vi "WS1050_VSA_Convert_Data Updated.vi"(6 "VSA_C3":string[][](array[string]), 7 "WS1050/51":bool=TRUE, 8 "error in (no error)":errorcluster, 9 "VSA_C2":string[][](array[string]), 10 "VSA_C1":string[][](array[string]), 11 "Voltage":string[][](array[string])) -> (0 "error out":errorcluster, 1 "VSA_V3":string[][](array[string]), 2 "VSA_V2":string[][](array[string]), 3 "VSA_V1":string[][](array[string]))   [LabVIEW 2012]
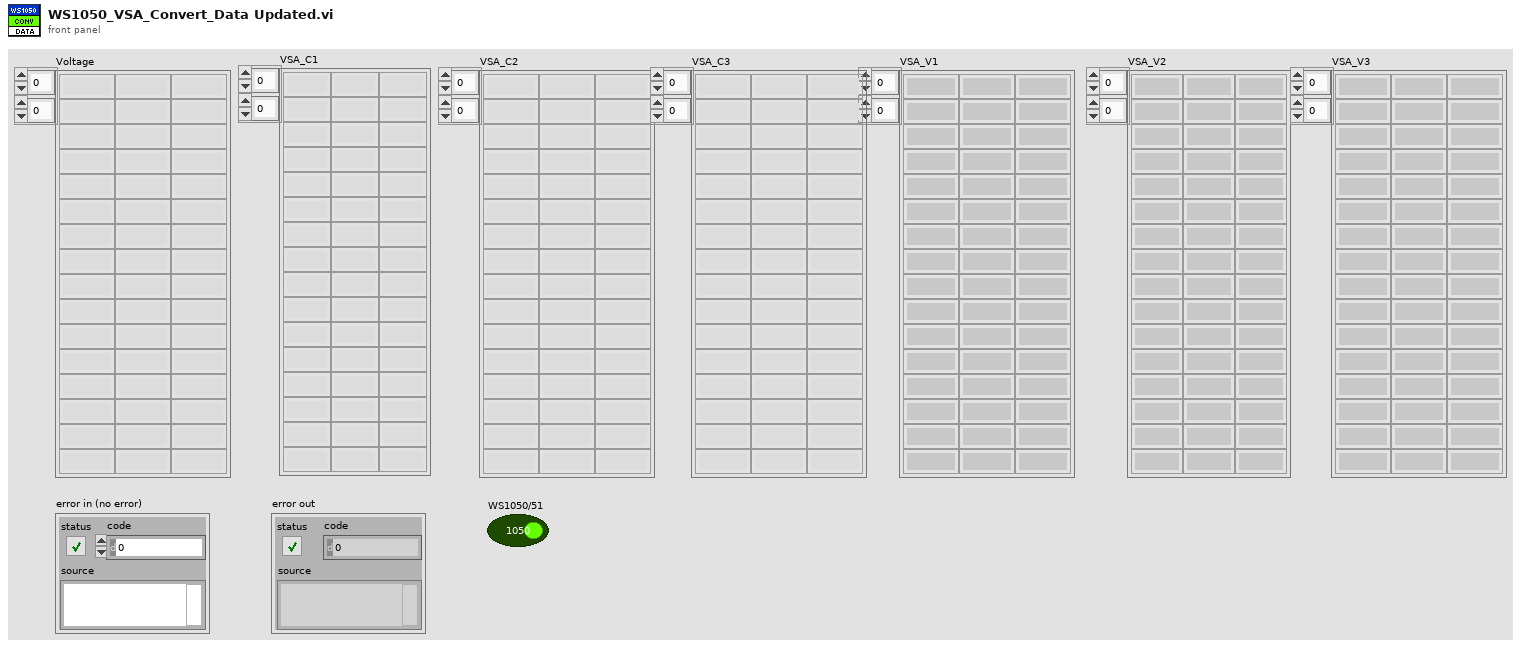
[diagram p1: front panel]
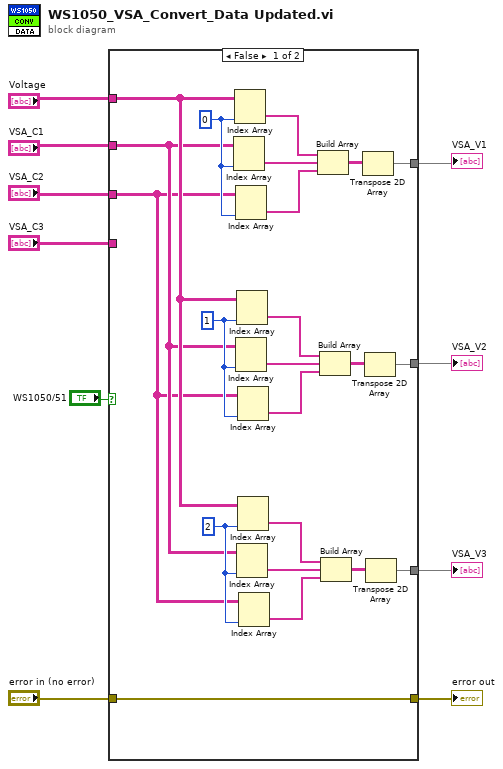
[diagram p0: block diagram]
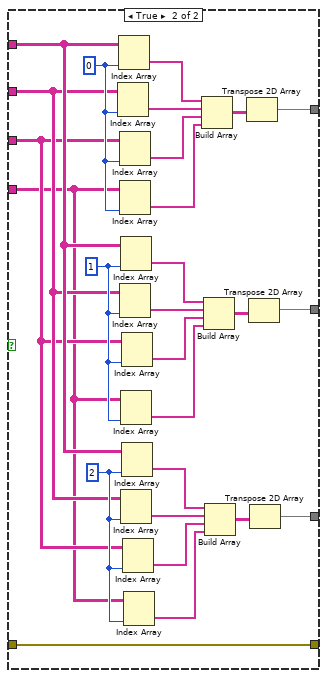
[diagram p2: hidden frame]
diagram:
  n1 = case shown="False" "WS1050/51" {
    tunnel: "error in (no error)" -> [w11 w58]
    tunnel: [w11 w58] -> w9
    tunnel: "Voltage" -> [w16 w57]
    tunnel: "VSA_C1" -> [w15 w38]
    tunnel: "VSA_C2" -> [w14 w37]
    tunnel: "VSA_C3" -> [_ w36]
    tunnel: [w17 w35] -> w3
    tunnel: [w12 w34] -> w2
    tunnel: [w13 w33] -> w1
    frame False {
      w18 = 2 ("disabled index (col)")
      w19 = 1 ("disabled index (col)")
      w20 = 0 ("disabled index (col)")
      n2 = Index Array(array=w15, index (col)=w20) -> (element=w31:string[])  [unwired: 1 in]
      n3 = Index Array(array=w16, index (col)=w20) -> (element=w32:string[])  [unwired: 1 in]
      n4 = Index Array(array=w14, index (col)=w20) -> (element=w30:string[])  [unwired: 1 in]
      n5 = Index Array(array=w15, index (col)=w19) -> (element=w26:string[])  [unwired: 1 in]
      n6 = Index Array(array=w16, index (col)=w19) -> (element=w25:string[])  [unwired: 1 in]
      n7 = Index Array(array=w15, index (col)=w18) -> (element=w23:string[])  [unwired: 1 in]
      n8 = Index Array(array=w14, index (col)=w19) -> (element=w27:string[])  [unwired: 1 in]
      n9 = Index Array(array=w16, index (col)=w18) -> (element=w24:string[])  [unwired: 1 in]
      n10 = Index Array(array=w14, index (col)=w18) -> (element=w22:string[])  [unwired: 1 in]
      n11 = Build Array(w32, w31, w30) -> (w29:string[][])
      n12 = Build Array(w25, w26, w27) -> (w28:string[][])
      n13 = Build Array(w24, w23, w22) -> (w21:string[][])
      n14 = Transpose 2D Array(2D array=w29) -> (transposed array=w17:string[][])
      n15 = Transpose 2D Array(2D array=w28) -> (transposed array=w12:string[][])
      n16 = Transpose 2D Array(2D array=w21) -> (transposed array=w13:string[][])
    }
    frame True {
      w40 = 2 ("disabled index (col)")
      w42 = 1 ("disabled index (col)")
      w44 = 0 ("disabled index (col)")
      n17 = Index Array(array=w38, index (col)=w44) -> (element=w55:string[])  [unwired: 1 in]
      n18 = Index Array(array=w57, index (col)=w44) -> (element=w56:string[])  [unwired: 1 in]
      n19 = Index Array(array=w37, index (col)=w44) -> (element=w54:string[])  [unwired: 1 in]
      n20 = Index Array(array=w36, index (col)=w44) -> (element=w43:string[])  [unwired: 1 in]
      n21 = Index Array(array=w38, index (col)=w42) -> (element=w50:string[])  [unwired: 1 in]
      n22 = Index Array(array=w57, index (col)=w42) -> (element=w49:string[])  [unwired: 1 in]
      n23 = Index Array(array=w36, index (col)=w42) -> (element=w41:string[])  [unwired: 1 in]
      n24 = Index Array(array=w38, index (col)=w40) -> (element=w47:string[])  [unwired: 1 in]
      n25 = Index Array(array=w37, index (col)=w42) -> (element=w51:string[])  [unwired: 1 in]
      n26 = Index Array(array=w57, index (col)=w40) -> (element=w48:string[])  [unwired: 1 in]
      n27 = Index Array(array=w37, index (col)=w40) -> (element=w46:string[])  [unwired: 1 in]
      n28 = Index Array(array=w36, index (col)=w40) -> (element=w39:string[])  [unwired: 1 in]
      n29 = Build Array(w56, w55, w54, w43) -> (w53:string[][])
      n30 = Build Array(w49, w50, w51, w41) -> (w52:string[][])
      n31 = Build Array(w48, w47, w46, w39) -> (w45:string[][])
      n32 = Transpose 2D Array(2D array=w53) -> (transposed array=w35:string[][])
      n33 = Transpose 2D Array(2D array=w52) -> (transposed array=w34:string[][])
      n34 = Transpose 2D Array(2D array=w45) -> (transposed array=w33:string[][])
    }
  }
  "error out" <- w9
  "VSA_V1" <- w3
  "VSA_V2" <- w2
  "VSA_V3" <- w1
